vi "PolyCommError.vi"   [LabVIEW 2011]
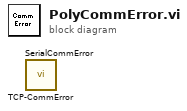
[diagram p0: block diagram]
diagram:
  n1 = call "TCP-CommError.vi"() -> ()  [unwired: 13 in, 3 out]
  n2 = call "SerialCommError.vi"() -> ()  [unwired: 13 in, 3 out]
